vi "Vision Processing.vi"(4 "error in (no error)":errorcluster, 5 "Camera Type":enum16{"206", "1011"}(ring)=enum."1011", 6 "Camera Name":string="Camera") -> ()   [LabVIEW 2011]
uses:
  Robot Global Data.vi
  <vilib>/vision/NI_Vision_Development_Module.lvlib
panel:
  in  "View":bool
  out "Target Info":T1(array[cluster])
  in  "Area Size Limit":i32=50
  in  "Particle Count Limit":i32=10
  in  "Score Limits":T2={"Rect Coverage"=76.0, "Aspect Ratio"=70.0, "X Edge Strength"=40.0, "Y Edge Strength"=60.0}
  in  "Processing":enum32{"Color", "Intensity", "Intensity Open"}(tab)=enum."Intensity"
  in  "Luminance":i32=125
  in  "Saturation":i32=60
  in  "Hue":i32(knob)=126 scale=0.0..255.0
  in  "Margins":cluster{"Hue":i32, "Sat":i32, "Lum":i32}={"Hue"=20, "Sat"=27, "Lum"=30} {"Sat" scale=0.0..40.0; "Lum" scale=0.0..40.0; "Hue" scale=0.0..40.0}
  in  "Range":cluster{"Lower value":sgl, "Upper value":sgl}={"Lower value"=150.0, "Upper value"=255.0} {"Lower value" scale=0.0..255.0; "Upper value" scale=0.0..255.0}
  in  "Range":cluster{"Lower value":sgl, "Upper value":sgl}={"Lower value"=150.0, "Upper value"=255.0} {"Lower value" scale=0.0..255.0; "Upper value" scale=0.0..255.0}
  in  "View":bool
  out "Processed Image":T3(plugin-control)
  # "Instructions:\nProcessing the reflective tape that is illuminated by a ring light can be based\non color or light intensity.\nParticles within the image are scored by rectangle coverage, aspect ratio, and\nfor being hollow with a bold edge. A particle is considered a target if all scores\nare above the score limits. Particles can be annotated -- surrounded by\na rectangle and scores drawn to the left .\nTo control the number of particles being scored, use the count limit and the size\nlimit."
  # "To debug, Enable using the View button.\nFor color processing, you can click in the image to select the color for processing."
  # "Enable by clicking the View button.\nGreen scores are above the limit, orange are below. Inner/outer rect\nindicates all passed."
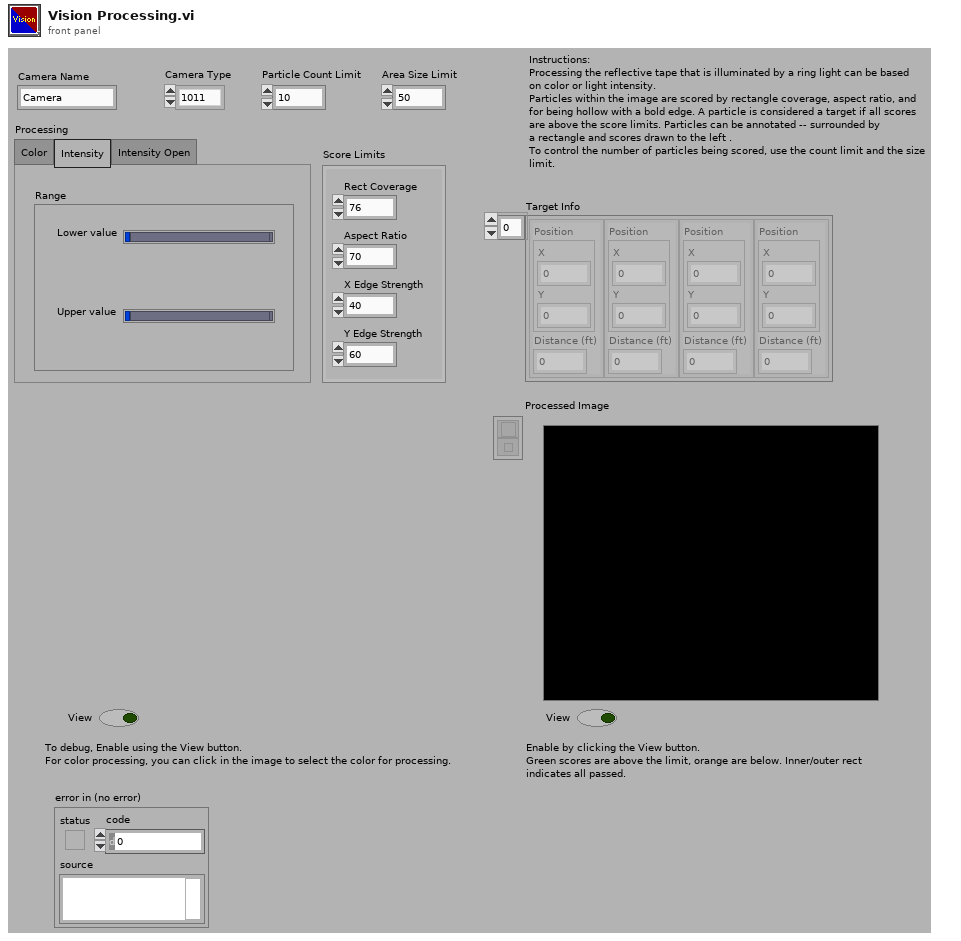
[diagram p1: front panel]
types:
  T1 = cluster{"Position":cluster{"X":dbl, "Y":dbl}, "Distance (ft)":dbl}[]
  T2 = cluster{"Rect Coverage":dbl, "Aspect Ratio":dbl, "X Edge Strength":dbl, "Y Edge Strength":dbl}
  T3 = typedef "IMAQ Image.ctl" = refnum<image>
  T4 = typedef "Image Type" = u32
  T5 = typedef "WPI_CameraDevRef.ctl" = cluster{"Camera Address":string, "CameraStatus":errorcluster, "Acquire Image Notifier":refnum<notifier>}
  T6 = enum32{"AutoM", "Close", "Dilate", "Erode", "Gradient", "Gradient out", "Gradient in", "Hit miss", "Open", "PClose", "POpen", "Thick", "Thin"}
  T7 = typedef "WPI_CameraImageSize.ctl" = enum16{"640x480", "320x240", "160x120"}
  T8 = cluster{cluster{"Left":dbl, "Top":dbl, "Right":dbl, "Bottom":dbl}, dbl[]}[]
  T9 = cluster{"Left":dbl, "Top":dbl, "Right":dbl, "Bottom":dbl}
  T10 = cluster{"Target Center (-1 to 1)":cluster{"X":dbl, "Y":dbl}, "Distance (ft)":dbl}
  T11 = cluster{"Target Center (-1 to 1)":cluster{"X":dbl, "Y":dbl}, "Distance (ft)":dbl}[]
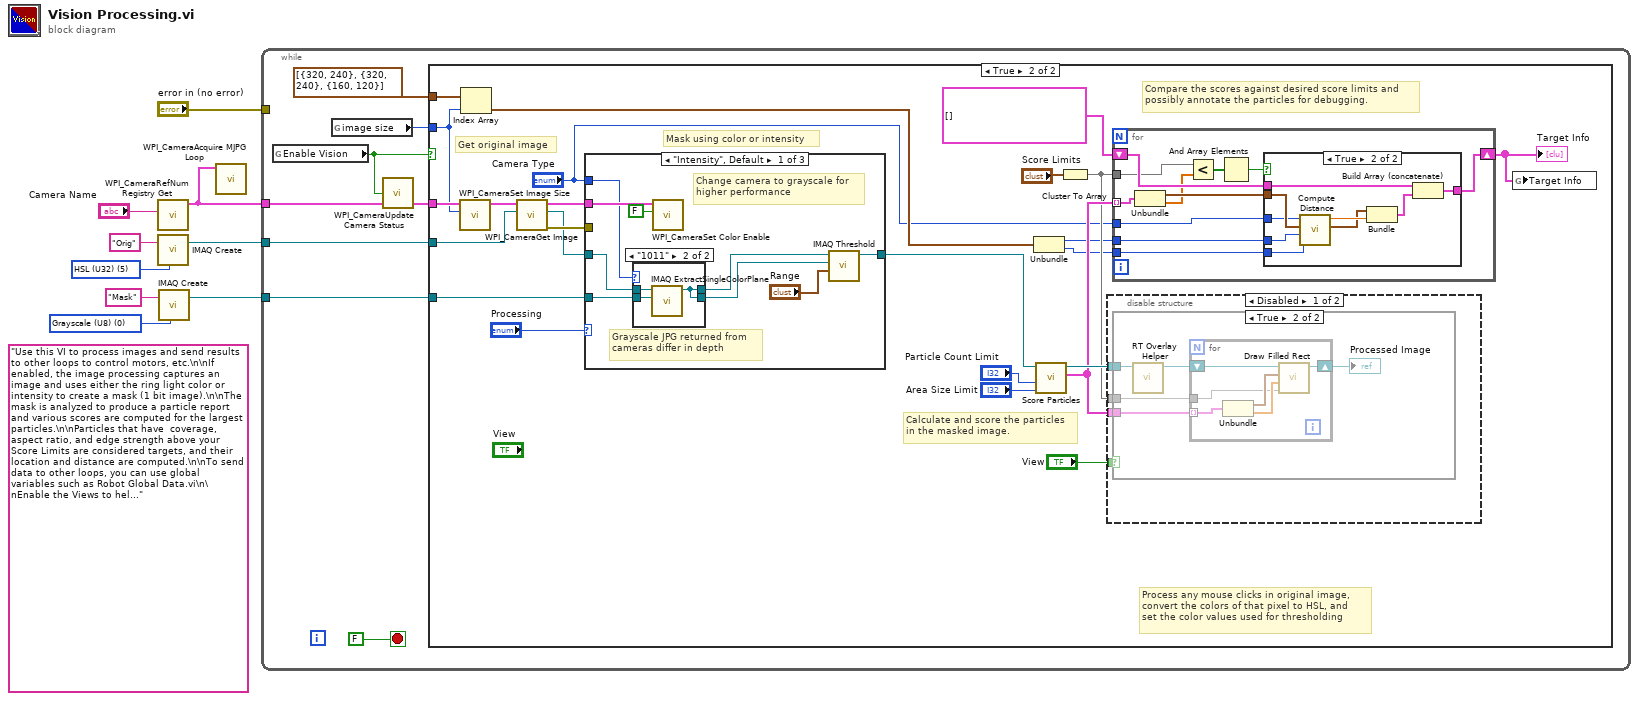
[diagram p0: block diagram]
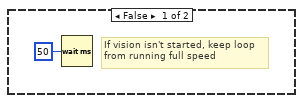
[diagram p2: hidden frame]
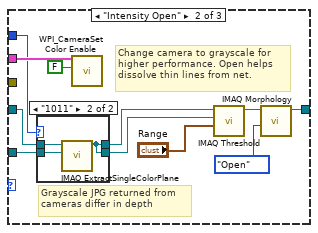
[diagram p6: hidden frame]
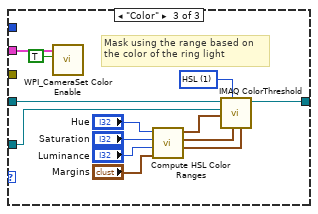
[diagram p8: hidden frame]
diagram:
  w3 = T4 0 items=["Grayscale (U8)", "Grayscale (I16)", "Grayscale (SGL)", "Complex (CSG)", "RGB (U32)", "HSL (U32)", "RGB (U64)", "Grayscale (U16)"] ("Image Type")
  (unwired) "Use this VI to process images and send results to other loops to control motors, etc.\n\nIf enabled, the image processing captures an image and uses either the ring light color or intensity to create a mask (1 bit image).\n\nThe mask is analyzed to produce a particle report and various scores are computed for the largest particles.\n\nParticles that have  coverage, aspect ratio, and edge strength above your Score Limits are considered targets, and their location and distance are computed.\n\nTo send data to other loops, you can use global variables such as Robot Global Data.vi\n\nEnable the Views to help debug color settings. Disable the View to speed up processing."
  w8 = T4 5 items=["Grayscale (U8)", "Grayscale (I16)", "Grayscale (SGL)", "Complex (CSG)", "RGB (U32)", "HSL (U32)", "RGB (U64)", "Grayscale (U16)"] ("Image Type")
  n1 = call <vilib>:"WPI_CameraRefNum Registry Get.vi"("refnum name"="Camera Name") -> ("CameraDevRef"=w5:T5)  [unwired: 9 in, 1 out]
  n2 = call "IMAQ Create"("Image Name"="Orig", "Image Type"=w8) -> ("New Image"=w7:T3)  [unwired: 2 in, 2 out]
  n3 = call "IMAQ Create"("Image Name"="Mask", "Image Type"=w3) -> ("New Image"=w1:T3)  [unwired: 2 in, 2 out]
  n4 = call <vilib>:"WPI_CameraAcquire MJPG Loop.vi"("CameraDevRef"=w5) -> ()  [unwired: 11 in]
  n5 = while {
    tunnel: w7 -> [w16]
    tunnel: w5 -> [w15]
    tunnel: "error in (no error)" -> [_]
    tunnel: w1 -> [w11]
    stop <- FALSE stop-if-true
    n6 = global read "Robot Global Data.vi" "Enable Vision"() -> (w13:bool)
    n7 = global read "Robot Global Data.vi" "image size"() -> (w12:T7)
    n8 = call <vilib>:"WPI_CameraUpdate Camera Status.vi"("CameraDevRef In"=w15, "Enable Vision"=w13) -> ("CameraDevRef Out"=w14:T5)  [unwired: 3 in]
    n9 = case shown="True" w13 {
      tunnel: w16 -> [_ w33]
      tunnel: w14 -> [_ w28]
      tunnel: w12 -> [_ w26]
      tunnel: w11 -> [_ w21]
      tunnel: cluster{i32, i32}[] [{320, 240}, {320, 240}, {160, 120}] -> [_ w25]
      frame False {
        # "If vision isn't started, keep loop\nfrom running full speed"
        n10 = Wait (ms)(milliseconds to wait=u32 50) -> ()  [unwired: 1 out]
      }
      frame True {
        # "Compare the scores against desired score limits and\npossibly annotate the particles for debugging."
        # "Process any mouse clicks in original image,\nconvert the colors of that pixel to HSL, and\nset the color values used for thresholding"
        # "Calculate and score the particles\nin the masked image."
        # "Mask using color or intensity"
        # "Get original image"
        n11 = call <vilib>:"WPI_CameraSet Image Size.vi"("Image Size"=w26, "CameraDevRef"=w28) -> ("CameraDevRef Out"=w29:T5)  [unwired: 8 in, 1 out]
        n12 = Index Array(array=w25, index=w26) -> (element=w22:cluster{i32, i32})
        n13 = call <vilib>:"WPI_CameraGet Image.vi"("Image"=w33, "CameraDevRef"=w29) -> ("error out"=w31:errorcluster, "Image Out"=w20:T3, "CameraDevRef Out"=w32:T5)  [unwired: 7 in]
        n14 = case shown="\"Intensity\", Default" "Processing" {
          tunnel: w20 -> [w62 w74 w100]
          tunnel: [w65 w79 w99] -> w27
          tunnel: w32 -> [w63 w77 w90]
          tunnel: w31 -> [_ _ _]
          tunnel: w21 -> [w61 w75 w88]
          tunnel: "Camera Type" -> [w60 w76 _]
          frame "Intensity", Default {
            # "Grayscale JPG returned from\ncameras differ in depth"
            # "Change camera to grayscale for\nhigher performance"
            n15 = case shown="\"1011\"" w60 {
              tunnel: w62 -> [w68 w71]
              tunnel: w61 -> [w67 w70]
              tunnel: [w68 w69] -> w59
              tunnel: [w67 w69] -> w58
              frame "206", Default {
              }
              frame "1011" {
                n16 = call "IMAQ ExtractSingleColorPlane"("Image Dst"=w70, "Image Src"=w71) -> ("Image Dst Out"=w69:T3)  [unwired: 8 in, 1 out]
              }
            }
            n17 = call <vilib>:"WPI_CameraSet Color Enable.vi"("Color Enabled"=FALSE, "CameraDevRef"=w63) -> ()  [unwired: 8 in, 2 out]
            n18 = call "IMAQ Threshold"("Range"="Range", "Image Dst"=w58, "Image Src"=w59) -> ("Image Dst Out"=w65:T3)  [unwired: 3 in, 5 out]
          }
          frame "Intensity Open" {
            # "Grayscale JPG returned from\ncameras differ in depth"
            # "Change camera to grayscale for\nhigher performance. Open helps\ndissolve thin lines from net."
            n19 = case shown="\"1011\"" w76 {
              tunnel: w74 -> [w84 w87]
              tunnel: w75 -> [w83 w86]
              tunnel: [w84 w85] -> w73
              tunnel: [w83 w85] -> w72
              frame "206", Default {
              }
              frame "1011" {
                n20 = call "IMAQ ExtractSingleColorPlane"("Image Dst"=w86, "Image Src"=w87) -> ("Image Dst Out"=w85:T3)  [unwired: 8 in, 1 out]
              }
            }
            n21 = call <vilib>:"WPI_CameraSet Color Enable.vi"("Color Enabled"=FALSE, "CameraDevRef"=w77) -> ()  [unwired: 8 in, 2 out]
            n22 = call "IMAQ Threshold"("Range"="Range", "Image Dst"=w72, "Image Src"=w73) -> ("Image Dst Out"=w80:T3)  [unwired: 3 in, 5 out]
            n23 = call "IMAQ Morphology"("Operation"=T6."Open", "Image Src"=w80) -> ("Image Dst Out"=w79:T3)  [unwired: 8 in, 1 out]
          }
          frame "Color" {
            w98 = u16 1 items=["RGB", "HSL", "HSV", "HSI"] ("Color Mode")
            # "Mask using the range based on\nthe color of the ring light"
            n24 = call <vilib>:"WPI_CameraSet Color Enable.vi"("Color Enabled"=TRUE, "CameraDevRef"=w90) -> ()  [unwired: 8 in, 2 out]
            n25 = call "Compute HSL Color Ranges.vi"("Margins"="Margins", "Luminance"="Luminance", "Saturation"="Saturation", "Hue"="Hue") -> ("Lum Range"=w95:cluster{i32, i32}, "Sat Range"=w96:cluster{i32, i32}, "Hue Range"=w97:cluster{i32, i32})  [unwired: 5 in]
            n26 = call "IMAQ ColorThreshold"("Blue or Luma or Val or Inten Range"=w95, "Green or Sat Range"=w96, "Color Mode"=w98, "Red or Hue Range"=w97, "Image Dst"=w88, "Image Src"=w100) -> ("Image Dst Out"=w99:T3)  [unwired: 4 in, 1 out]
          }
        }
        n27 = Unbundle(w22) -> (w24:i32, w23:i32)
        n28 = call "Score Particles.vi"("Area Size Limit"="Area Size Limit", "Particle Count Limit"="Particle Count Limit", "Image Refnum in"=w27) -> ("Scored Particle Info"=w38:T8, "Image Refnum out"=w41:T3)  [unwired: 7 in]
        n29 = Cluster To Array(cluster="Score Limits") -> (array=w36:dbl[])
        n30 = disable-structure shown="Disabled" {
          disable-tunnel: w41 -> [w46 _]
          disable-tunnel: w38 -> [w45 _]
          disable-tunnel: "View" -> [w44 _]
          disable-tunnel: w36 -> [w43 _]
          frame Disabled {
            n31 = case shown="True" w44 {
              tunnel: w46 -> [_ w48]
              tunnel: w45 -> [_ w50]
              tunnel: w43 -> [_ w49]
              frame False {
              }
              frame True {
                n32 = call "RT Overlay Helper.vi"("Refnum in"=w48) -> ("Refnum out"=w51:T3)  [unwired: 10 in]
                n33 = for {
                  shift-right: [w56] -> w47
                  shift-left: w51 -> [w57]
                  tunnel: w50 -> [w53] mode=indexing
                  tunnel: w49 -> [w52]
                  n34 = Unbundle(w53) -> (w54:T9, w55:dbl[])
                  n35 = call "Draw Filled Rect.vi"("Limits"=w52, "Scores"=w55, "Bounding Box"=w54, "image in"=w57) -> ("image out"=w56:T3)  [unwired: 7 in]
                }
                "Processed Image" <- w47
              }
            }
          }
          frame Enabled {
          }
        }
        n36 = for {
          shift-right: [w110] -> w30
          shift-left: T1 [] -> [w111]
          tunnel: w24 -> [w109]
          tunnel: w38 -> [w107] mode=indexing
          tunnel: w36 -> [w102]
          tunnel: "Camera Type" -> [w106]
          tunnel: w23 -> [w101]
          n37 = Unbundle(w107) -> (w108:T9, w103:dbl[])
          n38 = Less?(x=w102, y=w103) -> (x < y?=w105:bool[])
          n39 = And Array Elements(Boolean array=w105) -> (logical AND=w104:bool)
          n40 = case shown="True" w104 {
            tunnel: w111 -> [w112 w121]
            tunnel: [w112 w120] -> w110
            tunnel: w108 -> [_ w116]
            tunnel: w109 -> [_ w118]
            tunnel: w106 -> [_ w115]
            tunnel: w101 -> [_ w114]
            frame False {
            }
            frame True {
              n41 = call "Compute Distance.vi"("Y Image Resolution"=w114, "X Image Resolution"=w118, "Bounding Box"=w116, "Camera Type"=w115) -> ("Target Center (-1 to 1)"=w113:cluster{"X":dbl, "Y":dbl}, "Distance (ft)"=w117:dbl)  [unwired: 6 in]
              n42 = Bundle("Target Center (-1 to 1)"=w113, "Distance (ft)"=w117) -> (w119:T10)  [unwired: 1 in]
              n43 = Build Array (concatenate)(w121, w119) -> (w120:T11)
            }
          }
        }
        "Target Info" <- w30
        n44 = global write "Robot Global Data.vi" "Target Info"(w30) -> ()
      }
    }
  }
